vi "Configure Measurement Characteristics (Delta Time).vi"(0 "VISA resource name":refnum<visa-resource-name>, 1 "Stop Edge Direction (0: Rising)":i32(ring) items=["Rising", "Falling", "Either"], 2 "Stop Edge Position (1:Middle Level)":i32(ring)=1 items=["Upper Level", "Middle Level", "Lower Level"], 3 "Stop Edge Number (1)":i32=1, 5 "Start Edge Direction (0: Rising)":i32(ring) items=["Rising", "Falling", "Either"], 7 "Start Edge Position (1:Middle Level)":i32(ring)=1 items=["Upper Level", "Middle Level", "Lower Level"], 9 "Start Edge Number (1)":i32=1, 11 "error in (no error)":errorcluster) -> (4 "VISA resource name out":refnum<visa-resource-name>, 15 "error out":errorcluster)   [LabVIEW 2020, in "Agilent 90000 Series.lvlib"]
doc: "Defines the setup of delta time measurement, the number, direction and threshold of the start and stop edge that will be measured."
uses:
  Agilent 90000 Series.lvlib
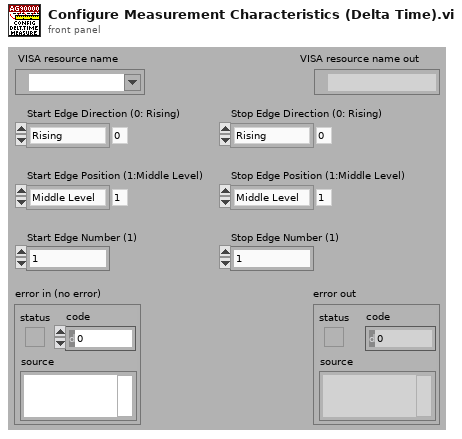
[diagram p1: front panel]
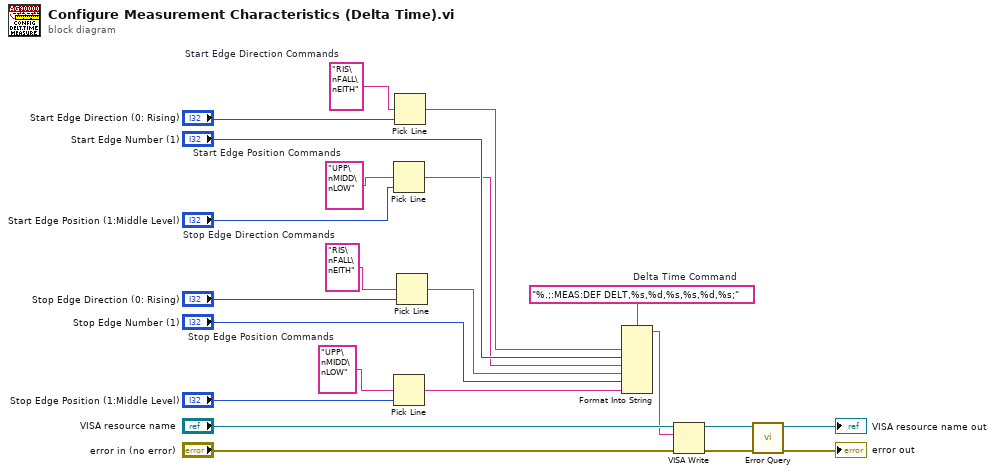
[diagram p0: block diagram]
diagram:
  w5 = "UPP\nMIDD\nLOW"  # Stop Edge Position Commands
  w9 = "RIS\nFALL\nEITH"  # Stop Edge Direction Commands
  w12 = "UPP\nMIDD\nLOW"  # Start Edge Position Commands
  w1 = "RIS\nFALL\nEITH"  # Start Edge Direction Commands
  w16 = "%.;:MEAS:DEF DELT,%s,%d,%s,%s,%d,%s;"  # Delta Time Command
  n1 = Pick Line(multi-line string=w12, line index="Start Edge Position (1:Middle Level)") -> (output string=w10:string)  [unwired: 1 out]
  n2 = Pick Line(multi-line string=w5, line index="Stop Edge Position (1:Middle Level)") -> (output string=w3:string)  [unwired: 1 out]
  n3 = Pick Line(multi-line string=w1, line index="Start Edge Direction (0: Rising)") -> (output string=w14:string)  [unwired: 1 out]
  n4 = Pick Line(multi-line string=w9, line index="Stop Edge Direction (0: Rising)") -> (output string=w7:string)  [unwired: 1 out]
  n5 = Format Into String(format string=w16, w14, "Start Edge Number (1)", w10, w7, "Stop Edge Number (1)", w3) -> (resulting string=w2:string)  [unwired: 2 in, 1 out]
  n6 = VISA Write(VISA resource name="VISA resource name", write buffer=w2, error in (no error)="error in (no error)") -> (VISA resource name out=w18:refnum<visa-resource-name>, error out=w17:errorcluster)  [unwired: 1 out]
  n7 = call "Error Query.vi"("error in (no error)"=w17, "VISA resource name"=w18) -> ("error out"=→"error out":errorcluster, "VISA resource name out"=→"VISA resource name out":refnum<visa-resource-name>)  [unwired: 8 out]
